vi "Launcher.vi"   [LabVIEW 2019]
uses:
  507e2b93-ff01-48ad-8c07-dd2eea017277.vi
  Libraries/Audio Input/Audio Input.lvlib
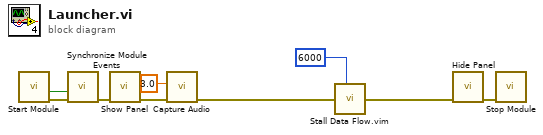
[diagram p0: block diagram]
diagram:
  n1 = call "Start Module.vi"() -> ("error out"=w9:errorcluster, "Wait for Event Sync?"=w6:bool)  [unwired: 8 in, 2 out]
  n2 = call "Synchronize Module Events.vi"("error in (no error)"=w9, "Wait for Event Sync?"=w6) -> ("error out"=w8:errorcluster)  [unwired: 9 in]
  n3 = call "Show Panel.vi"("error in (no error)"=w8) -> ("error out"=w3:errorcluster)  [unwired: 10 in]
  n4 = call "Capture Audio.vi"("error in (no error)"=w3, "Capture Time (s)(2)"=3.0) -> ("error out"=w2:errorcluster)  [unwired: 9 in]
  n5 = call "Stall Data Flow.vim"("value in"=w2, "milliseconds to wait"=u32 6000) -> ("value out"=w5:errorcluster)  [unwired: 1 out]
  n6 = call "Hide Panel.vi"("error in (no error)"=w5) -> ("error out"=w7:errorcluster)  [unwired: 10 in]
  n7 = call "Stop Module.vi"("error in (no error)"=w7) -> ()  [unwired: 10 in, 1 out]
